vi "thermocouples.vi"() -> ()   [LabVIEW 2025]
uses:
  Classes/Thermocouples/Thermocouples.lvclass
panel:
  out "Waveform Chart":T1(graph)
  in  "stop":bool
  out "Temps":dbl[](array[numeric]) format="%0.2f"
  out "error out 2":errorcluster
  out "Thermocouples out":refnum<class "Thermocouples.lvclass">
  out "error out":errorcluster
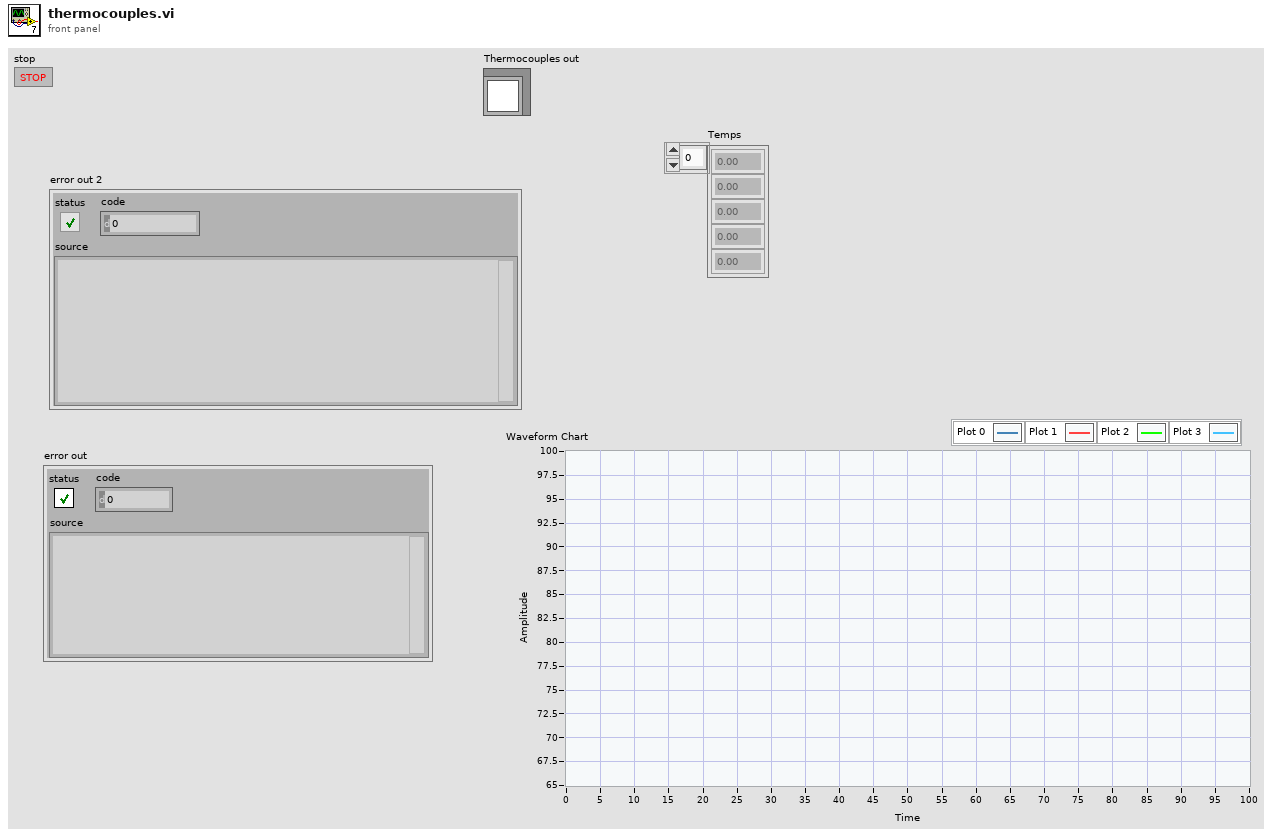
[diagram p1: front panel]
types:
  T1 = cluster{"Temps[0]":dbl, "Temps[1]":dbl, "Temps[2]":dbl, "Temps[3]":dbl, "Temps[4]":dbl, "Temps[5]":dbl, "Temps[6]":dbl, "Temps[7]":dbl, "Temps[8]":dbl}
  T2 = cluster{"Thermocouples":refnum<class "Thermocouples.lvclass">, "Relays":refnum<class "Relays.lvclass">}
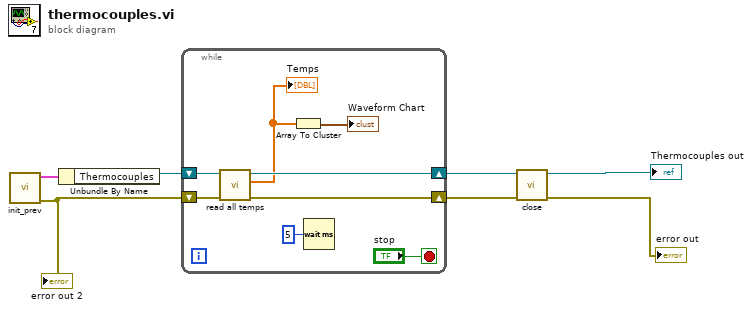
[diagram p0: block diagram]
diagram:
  n1 = call "init_prev.vi"() -> ("error out"=w3:errorcluster, "output cluster"=w6:T2)  [unwired: 10 in]
  "error out 2" <- w3
  n2 = Unbundle By Name(w6) -> ("Thermocouples"=w4:refnum<class "Thermocouples.lvclass">)
  n3 = while {
    shift-right: [w13] -> w2
    shift-left: w4 -> [w15]
    shift-right: [w12] -> w1
    shift-left: w3 -> [w14]
    stop <- "stop" stop-if-true
    n4 = call-dynamic "read all temps.vi"("error in (no error)"=w14, "Thermocouples in"=w15) -> ("error out"=w12:errorcluster, "Temps"=w9:dbl[], "Thermocouples out"=w13:refnum<class "Thermocouples.lvclass">)  [unwired: 7 in]
    "Temps" <- w9
    n5 = Array To Cluster(array=w9) -> (cluster=→"Waveform Chart":T1)
    n6 = Wait (ms)(milliseconds to wait=u32 5) -> ()  [unwired: 1 out]
  }
  n7 = call-dynamic "close.vi"("error in (no error)"=w1, "Thermocouples in"=w2) -> ("error out"=→"error out":errorcluster, "Thermocouples out"=→"Thermocouples out":refnum<class "Thermocouples.lvclass">)  [unwired: 8 in]
